vi "Hardware-DI-B Sim Settings-Host.vi"() -> ()   [LabVIEW 2016]
panel:
  in  "PumpCapacitance":sgl=5e-06 caption="[Farad]" format="%#_6p"
  in  "PumpInductance":sgl=0.0001 caption="[Henry]" format="%#_6p"
  in  "PumpResistance":sgl=1.0 caption="[]" format="%#_6p"
  in  "InjCapacitance":sgl=5e-06 caption="[]" format="%#_6p"
  in  "InjInductance":sgl=0.0001 caption="[]" format="%#_6p"
  in  "InjResistance":sgl=1.0 caption="[]" format="%#_6p"
  in  "SimRotations":u8=1 caption="[]"
  in  "SimSpeed":sgl=3000.0 caption="[]"
  in  "SimBatt":sgl=13.7 caption="[]"
  # "DI-B Injector and Pump Simulation \nSettings"
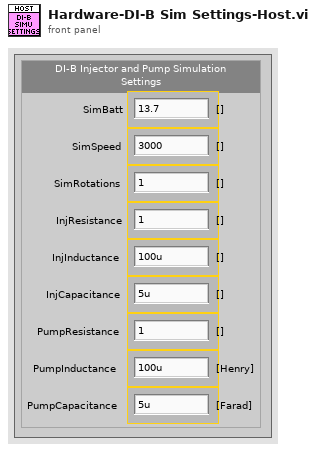
[diagram p1: front panel]
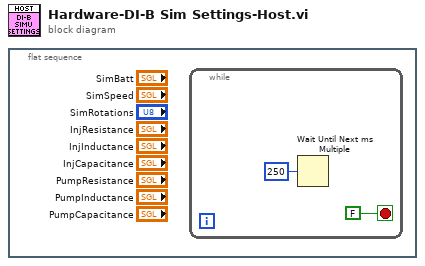
[diagram p0: block diagram]
diagram:
  n1 = flat-sequence {
    frame #0 {
      n2 = while {
        stop <- FALSE stop-if-true
        n3 = Wait Until Next ms Multiple(millisecond multiple=u32 250) -> ()  [unwired: 1 out]
      }
    }
  }
